vi "FindBrackets.vi"(1 "String in":string) -> (0 "String out":string)   [LabVIEW 2019]
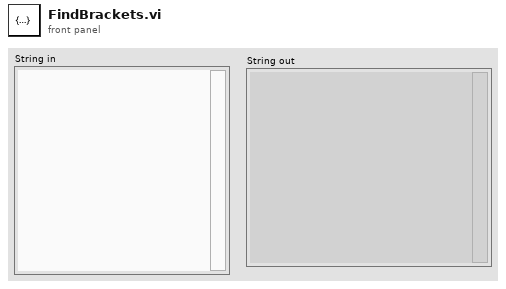
[diagram p1: front panel]
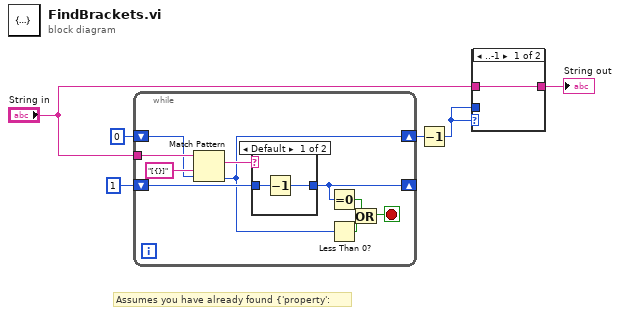
[diagram p0: block diagram]
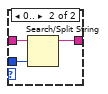
[diagram p2: hidden frame]
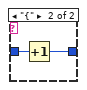
[diagram p3: hidden frame]
diagram:
  # "Assumes you have already found {'property':"
  n1 = while {
    tunnel: "String in" -> [w15]
    shift-right: [w10] -> w4
    shift-left: 0 ("offset past match") -> [w14]
    shift-right: [w11] -> _
    shift-left: 1 -> [w12]
    stop <- w7 stop-if-true
    n2 = Match Pattern(string=w15, regular expression="[{}]", offset (0)=w14) -> (match substring=w13:string, offset past match=w10:i32)  [unwired: 2 out]
    n3 = case shown="Default" w13 {
      tunnel: w12 -> [w18 w20]
      tunnel: [w17 w19] -> w11
      frame Default {
        n4 = Decrement(x=w18) -> (x-1=w17:i32)
      }
      frame "{" {
        n5 = Increment(x=w20) -> (x+1=w19:i32)
      }
    }
    n6 = Equal To 0?(x=w11) -> (x = 0?=w8:bool)
    n7 = Less Than 0?(x=w10) -> (x < 0?=w9:bool)
    n8 = Or(x=w8, y=w9) -> (x .or. y?=w7:bool)
  }
  n9 = Decrement(x=w4) -> (x-1=w6:i32)
  n10 = case shown="..-1" w6 {
    tunnel: "String in" -> [w21 w24]
    tunnel: [w21 w23] -> w5
    tunnel: w6 -> [_ w22]
    frame ..-1 {
    }
    frame 0.. {
      n11 = Search/Split String(string=w24, offset (0)=w22) -> (substring before match=w23:string)  [unwired: 1 in, 2 out]
    }
  }
  "String out" <- w5
